vi "RunServo (1).vi"() -> ()   [LabVIEW 2018]
uses:
  <vilib>/myRIO/Common/Instrument Driver Framework/myRIO v1.0/PWM/vis/myRIO v1.1 Open PWM.vi
  <vilib>/myRIO/Common/Instrument Driver Framework/myRIO v1.0/UART/vis/myRIO v1.0 Close UART.vi
  <vilib>/myRIO/Common/Instrument Driver Framework/Utilities/vis/Validate Channels.vi
  <vilib>/myRIO/Common/Instrument Driver Framework/myRIO v1.0/PWM/vis/myRIO v1.0 Reserve PWM.vi
  <vilib>/myRIO/Common/Instrument Driver Framework/myRIO v1.0/PWM/vis/myRIO v1.0 Build MUX Configuration PWM.vi
  <vilib>/myRIO/Common/Instrument Driver Framework/myRIO v1.0/Resource Manager/vis/myRIO v1.0 Reserve Channel List.vi
  <vilib>/myRIO/Common/Instrument Driver Framework/myRIO v1.0/Resource Manager/vis/myRIO v1.0 Create Configuration List.vi
  <vilib>/myRIO/Common/Instrument Driver Framework/myRIO v1.0/Resource Manager/vis/myRIO v1.0 Reserve Channel.vi
  <vilib>/myRIO/Common/Instrument Driver Framework/myRIO v1.0/Resource Manager/vis/myRIO v1.0 Unreserve Channel.vi
  <vilib>/myRIO/Common/Instrument Driver Framework/myRIO v1.0/Resource Manager/vis/myRIO v1.0 Build Mutex Name.vi
  <vilib>/Utility/VariantDataType/GetNumericInfo.vi
  <vilib>/Utility/error.llb/Error Cluster From Error Code.vi
  <vilib>/myRIO/Common/Instrument Driver Framework/myRIO v1.0/myRIO v1.1 Open.vi
  <vilib>/myRIO/Common/Instrument Driver Framework/Utilities/vis/IO Manager.vi
  <vilib>/myRIO/Common/Instrument Driver Framework/Utilities/vis/Configuration Manager.vi
  <vilib>/myRIO/Common/Instrument Driver Framework/myRIO v1.0/Resource Manager/vis/myRIO v1.0 Configure IO.vi
  <vilib>/myRIO/Common/Instrument Driver Framework/myRIO v1.0/myRIO v1.0 Close.vi
  <vilib>/myRIO/Common/Instrument Driver Framework/myRIO v1.0/PWM/vis/myRIO v1.0 Write PWM.vi
  <vilib>/myRIO/Common/Instrument Driver Framework/Utilities/vis/FPGA Ref Manager.vi
  <vilib>/myRIO/Common/Instrument Driver Framework/myRIO v1.0/myRIO v1.0 Reset FPGA.vi
  <vilib>/myRIO/Common/Instrument Driver Framework/myRIO v1.0/IRQ/vis/myRIO v1.0 IRQ Info FGV.vi
  <vilib>/myRIO/Common/Instrument Driver Framework/myRIO v1.0/IRQ/vis/myRIO v1.0 Timer IRQ Info FGV.vi
  <vilib>/myRIO/Common/Instrument Driver Framework/myRIO v1.0/IRQ/vis/myRIO v1.0 ISR Agent.vi
  <vilib>/myRIO/Instrument Drivers/Utilities/Utilities.lvlib
  <vilib>/myRIO/Instrument Drivers/Onboard IO/PWM/PWM.lvlib
panel:
  out "Cloud Value":dbl
  out "offset [%FS] 2":dbl
  out "duty cycle [%] 2":dbl
  out "pulse width [ms] 2":dbl=1.5
  in  "freq [Hz] 2":dbl=50.0
  in  "position [%FS] 2":dbl(slide) scale=-200.0..200.0
  in  "PWM channel 2":tag="B/PWM0"
  out "offset [%FS]":dbl
  out "duty cycle [%]":dbl
  out "pulse width [ms]":dbl=1.5
  in  "freq [Hz]":dbl=50.0
  in  "PWM channel":tag="B/PWM0"
  in  "[ESC]":bool
  # "Servo2"
  # "Servo1"
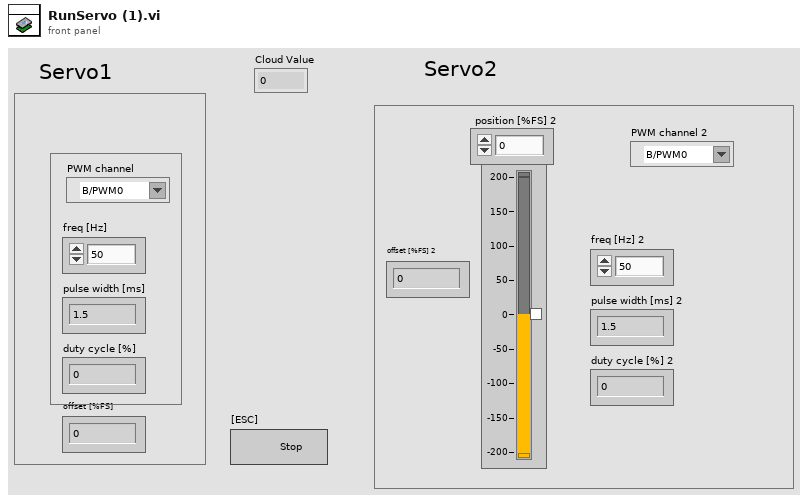
[diagram p1: front panel]
types:
  T1 = typedef "PWM.lvlib/PWM Reference.ctl" = cluster{"myRIO Reference":T2, "PWM Channels Enum":T6, "PWM Configuration":T7}
  T2 = typedef "myRIO Generic Hardware Reference.ctl" = cluster{"myRIO Model":T3, "myRIO Hardware Reference":T4}
  T3 = typedef "Hardware Version Enum.ctl" = enum16{"Unknown", "myRIO-1900", "myRIO-1950", "roboRIO", "NI ELVIS RIO CM", "ELVIS III"}
  T4 = typedef "myRIO v1.0 Reference.ctl" = cluster{"Generic FPGA Reference":T5, "Allow multiple opens":bool}
  T5 = typedef "Generic FPGA Reference.ctl" = refnum<k20>
  T6 = typedef "PWM Channels Enum.ctl" = enum16{"Not Connected", "C/PWM0", "C/PWM1", "A/PWM0", "A/PWM1", "A/PWM2", "A/PWM3", "A/PWM4", "A/PWM5", "A/PWM6", "A/PWM7", "A/PWM8", "A/PWM9", "A/PWM10", "A/PWM11", "A/PWM12", "A/PWM13", "A/PWM14", "A/PWM15", "A/PWM16", "A/PWM17", "A/PWM18", "A/PWM19", "B/PWM0", "B/PWM1", "B/PWM2", "B/PWM3", "B/PWM4", "B/PWM5", "B/PWM6", "B/PWM7", "B/PWM8", "B/PWM9", "B/PWM10", "B/PWM11", "B/PWM12", "B/PWM13", "B/PWM14", "B/PWM15", "B/PWM16", "B/PWM17", "B/PWM18", "B/PWM19", "PWM/PWM0", "PWM/PWM1", "PWM/PWM2", "PWM/PWM3", "PWM/PWM4", "PWM/PWM5", "PWM/PWM6", "PWM/PWM7", "PWM/PWM8", "PWM/PWM9"}
  T7 = typedef "PWM.lvlib/PWM Configuration.ctl" = cluster{"Frequency":dbl, "Duty Cycle":dbl}
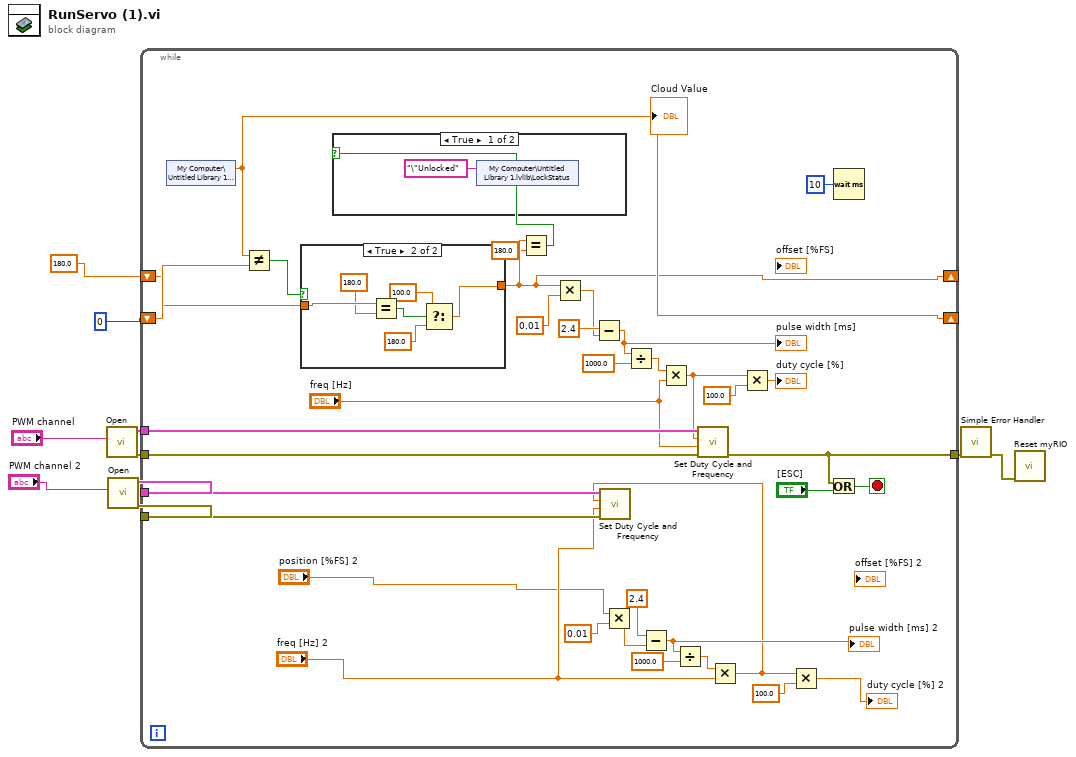
[diagram p0: block diagram]
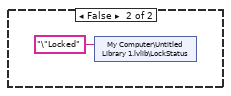
[diagram p2: hidden frame]
diagram:
  n1 = call <vilib>:"Open.vi"("Channel Name"="PWM channel") -> ("error out"=w7:errorcluster, "PWM Ref Out"=w8:T1)  [unwired: 9 in]
  n2 = call <vilib>:"Open.vi"("Channel Name"="PWM channel 2") -> ("error out"=w3:errorcluster, "PWM Ref Out"=w4:T1)  [unwired: 9 in]
  n3 = while {
    tunnel: w8 -> [w40]
    tunnel: w7 -> [w39]
    tunnel: [w38] -> w6
    tunnel: w4 -> [w34]
    tunnel: w3 -> [w33]
    shift-right: [w14] -> _
    shift-left: 0 -> [w17]
    shift-right: [w13] -> _
    shift-left: 180.0 ("f") -> [w15]
    stop <- w46 stop-if-true
    n4 = shared-variable "My Computer\\Untitled Library 1.lvlib\\RFID"() -> (w14:dbl)  [unwired: 1 in, 1 out]
    "Cloud Value" <- w14
    n5 = Not Equal?(x=w14, y=w17) -> (x != y?=w16:bool)
    n6 = case shown="True" w16 {
      tunnel: w15 -> [w49 w55]
      tunnel: [w49 w50] -> w13
      frame False {
      }
      frame True {
        n7 = Equal?(x=w55, y=180.0 ("f")) -> (x = y?=w53:bool)
        n8 = Select(t=100.0, s=w53, f=180.0) -> (s? t:f=w50:dbl)
      }
    }
    n9 = Equal?(x=w13, y=180.0) -> (x = y?=w11:bool)
    n10 = case shown="True" w11 {
      frame True {
        n11 = shared-variable "My Computer\\Untitled Library 1.lvlib\\LockStatus"("\"Unlocked" ("LockStatus")) -> ()  [unwired: 1 in, 1 out]
      }
      frame False {
        n12 = shared-variable "My Computer\\Untitled Library 1.lvlib\\LockStatus"("\"Locked" ("LockStatus")) -> ()  [unwired: 1 in, 1 out]
      }
    }
    n13 = Multiply(x=w13, y=0.01) -> (x*y=w20:dbl)
    n14 = Subtract(x=2.4 ("y"), y=w20) -> (x-y=w42:dbl)
    "pulse width [ms]" <- w42
    n15 = Multiply(x="position [%FS] 2", y=0.01) -> (x*y=w18:dbl)
    n16 = Divide(x=w42, y=1000.0) -> (x/y=w37:dbl)
    n17 = Subtract(x=2.4 ("y"), y=w18) -> (x-y=w26:dbl)
    "pulse width [ms] 2" <- w26
    n18 = Multiply(x=w37, y="freq [Hz]") -> (x*y=w31:dbl)
    n19 = Divide(x=w26, y=1000.0) -> (x/y=w28:dbl)
    n20 = call <vilib>:"Set Duty Cycle and Frequency.vi"("error in (no error)"=w39, "Frequency [Hz]"="freq [Hz]", "Duty Cycle"=w31, "PWM Ref In"=w40) -> ("error out"=w38:errorcluster)  [unwired: 5 in, 1 out]
    n21 = Multiply(x=w28, y="freq [Hz] 2") -> (x*y=w23:dbl)
    n22 = call <vilib>:"Set Duty Cycle and Frequency.vi"("error in (no error)"=w33, "Frequency [Hz]"="freq [Hz] 2", "Duty Cycle"=w23, "PWM Ref In"=w34) -> ()  [unwired: 5 in, 2 out]
    n23 = Multiply(x=w31, y=100.0) -> (x*y=→"duty cycle [%]":dbl)
    n24 = Multiply(x=w23, y=100.0) -> (x*y=→"duty cycle [%] 2":dbl)
    n25 = Or(x=w38, y="[ESC]") -> (x .or. y?=w46:bool)
    n26 = Wait (ms)(milliseconds to wait=u32 10) -> ()  [unwired: 1 out]
  }
  n27 = call <vilib>:"Simple Error Handler.vi"("error in (no error)"=w6) -> ("error out"=w10:errorcluster)  [unwired: 4 in, 4 out]
  n28 = call <vilib>:"Reset myRIO.vi"("error in (no error)"=w10) -> ()  [unwired: 10 in, 1 out]
